vi "Finish.vi"   [LabVIEW 2018]
doc: "This VI is called just before exiting. It is expected to close I/O refnum, save collected data, etc."
uses:
  <vilib>/Rock Robotics/WPI/Utilities/WPI_GetSetVariantRefNum.vi
types:
  T1 = typedef "WPI_MotorControlDeviceRef.ctl" = cluster{"DeviceStatus":errorcluster, "Type":T2, "PWM":cluster{"PWM Channel":T3, "DeadBand":T4}, "CAN":cluster{"Device Number":u8, "SetOutput VI Ref":variant, "GetOutput VI Ref":variant, "Enable VI Ref":variant, "Disable VI Ref":variant, "Data":variant}, "Invert":bool, "DIO PWM":cluster{"PWM \"Enable\" Channel":T3, "DIOChannel":T5, "PWM Rate":dbl}}
  T2 = typedef "WPI_MotorControlType.ctl" = enum16{"PWM", "CAN", "DIO PWM"}
  T3 = typedef "FPGA_DIOPWMChannel.ctl" = enum8{"PWM 0", "PWM 1", "PWM 2", "PWM 3", "PWM 4", "PWM 5", "PWM 6", "PWM 7", "PWM 8", "PWM 9", "PWM MXP 0", "PWM MXP 1", "PWM MXP 2", "PWM MXP 3", "PWM MXP 4", "PWM MXP 5", "PWM MXP 6", "PWM MXP 7", "PWM MXP 8", "PWM MXP 9", "Invalid"}
  T4 = typedef "WPI_PWMDeadband.ctl" = cluster{"Name":string, "maxPositivePwm":i32, "minPositivePwm":i32, "centerPwm":i32, "maxNegativePwm":i32, "minNegativePwm":i32, "angularRange":u16}
  T5 = typedef "FPGA_DIOChannel.ctl" = enum8{"DIO 0", "DIO 1", "DIO 2", "DIO 3", "DIO 4", "DIO 5", "DIO 6", "DIO 7", "DIO 8", "DIO 9", "DIO MXP 0", "DIO MXP 1", "DIO MXP 2", "DIO MXP 3", "DIO MXP 4", "DIO MXP 5", "DIO MXP 6", "DIO MXP 7", "DIO MXP 8", "DIO MXP 9", "DIO MXP 10", "DIO MXP 11", "DIO MXP 12", "DIO MXP 13", "DIO MXP 14", "DIO MXP 15", "SPI Port CS1", "SPI Port CS2", "SPI Port CS3", "SPI Port MISO", "SPI Port MOSI", "Invalid"}
  T6 = typedef "WPI_SolenoidDevRef.ctl" = cluster{"DevStatus":errorcluster, "Pneumatics Control Module":u8, "Forward Solenoid Channel":T7, "Reverse Solenoid Channel":T7}
  T7 = typedef "WPI_SolenoidChannel.ctl" = enum8{"Solenoid 0", "Solenoid 1", "Solenoid 2", "Solenoid 3", "Solenoid 4", "Solenoid 5", "Solenoid 6", "Solenoid 7", "Invalid"}
  T8 = typedef "WPI_SwitchDevRef.ctl" = cluster{"DevStatus":errorcluster, "DIO Channel":T5, "CntIndex":T9, "Normally Closed":bool}
  T9 = typedef "FPGA_CounterCtrSystemIndex.ctl" = enum8{"Ctr 0", "Ctr 1", "Ctr 2", "Ctr 3", "Ctr 4", "Ctr 5", "Ctr 6", "Ctr 7", "Invalid"}
  T10 = typedef "WPI_JoystickDevRef.ctl" = cluster{"Device":T11}
  T11 = typedef "WPI_JoystickDeviceEnum.ctl" = enum16{"USB 0", "USB 1", "USB 2", "USB 3", "USB 4", "USB 5"}
  T12 = typedef "WPI_RobotDriveDevRef.ctl" = cluster{"DevStatus":errorcluster, "Motors[]":T1[], "Square Inputs":bool, "Max Output":dbl}
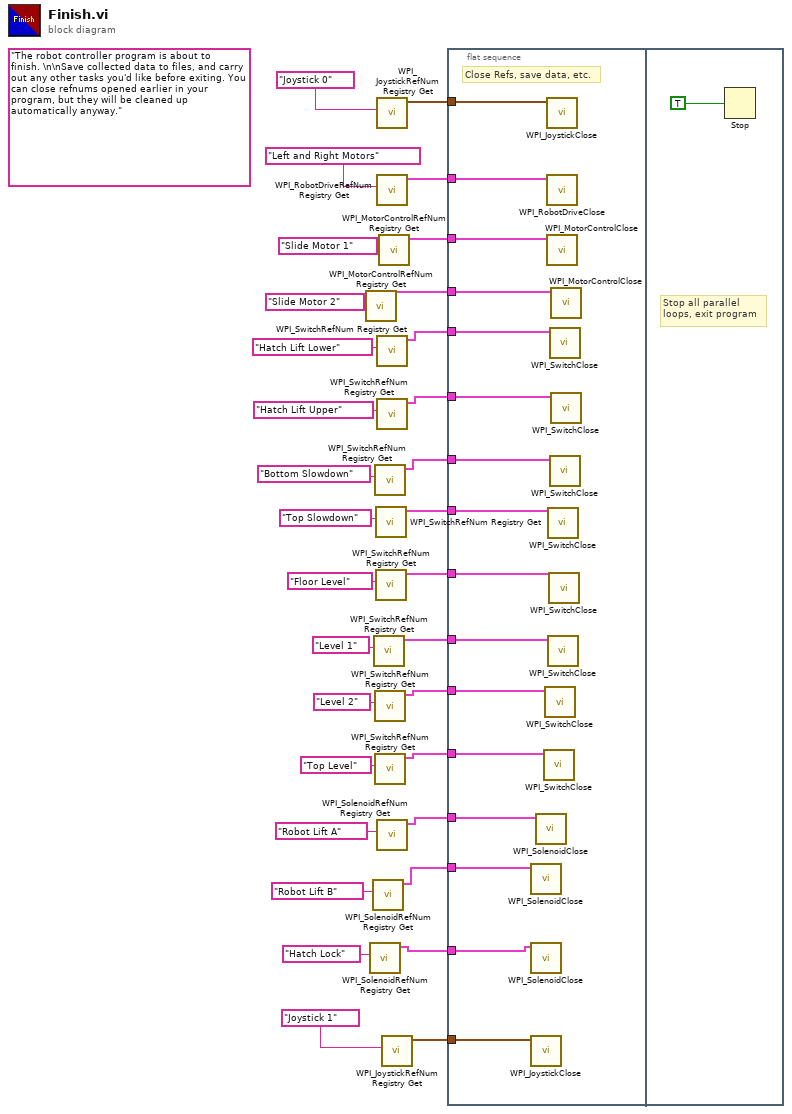
[diagram p0: block diagram]
diagram:
  (unwired) "The robot controller program is about to finish. \n\nSave collected data to files, and carry out any other tasks you'd like before exiting. You can close refnums opened earlier in your program, but they will be cleaned up automatically anyway."
  n1 = call <vilib>:"WPI_MotorControlRefNum Registry Get.vi"("refnum name"="Slide Motor 2") -> ("MotorControlDevRef"=w19:T1)  [unwired: 9 in, 1 out]
  n2 = call <vilib>:"WPI_SolenoidRefNum Registry Get.vi"("refnum name"="Hatch Lock") -> ("SolenoidDevRef"=w3:T6)  [unwired: 9 in, 1 out]
  n3 = call <vilib>:"WPI_SolenoidRefNum Registry Get.vi"("refnum name"="Robot Lift B") -> ("SolenoidDevRef"=w4:T6)  [unwired: 9 in, 1 out]
  n4 = call <vilib>:"WPI_SwitchRefNum Registry Get.vi"("refnum name"="Level 1") -> ("SwitchDevRef"=w24:T8)  [unwired: 9 in, 1 out]
  n5 = call <vilib>:"WPI_SwitchRefNum Registry Get.vi"("refnum name"="Bottom Slowdown") -> ("SwitchDevRef"=w11:T8)  [unwired: 9 in, 1 out]
  n6 = call <vilib>:"WPI_SwitchRefNum Registry Get.vi"("refnum name"="Level 2") -> ("SwitchDevRef"=w13:T8)  [unwired: 9 in, 1 out]
  n7 = call <vilib>:"WPI_SwitchRefNum Registry Get.vi"("refnum name"="Top Level") -> ("SwitchDevRef"=w12:T8)  [unwired: 9 in, 1 out]
  n8 = call <vilib>:"WPI_SwitchRefNum Registry Get.vi"("refnum name"="Top Slowdown") -> ("SwitchDevRef"=w28:T8)  [unwired: 9 in, 1 out]
  n9 = call <vilib>:"WPI_SwitchRefNum Registry Get.vi"("refnum name"="Floor Level") -> ("SwitchDevRef"=w25:T8)  [unwired: 9 in, 1 out]
  n10 = call <vilib>:"WPI_JoystickRefNum Registry Get.vi"("refnum name"="Joystick 0") -> ("JoystickDevRef"=w29:T10)  [unwired: 1 in, 9 out]
  n11 = call <vilib>:"WPI_RobotDriveRefNum Registry Get.vi"("refnum name"="Left and Right Motors") -> ("RobotDriveDevRef"=w30:T12)  [unwired: 1 in, 9 out]
  n12 = call <vilib>:"WPI_SwitchRefNum Registry Get.vi"("refnum name"="Hatch Lift Lower") -> ("SwitchDevRef"=w9:T8)  [unwired: 9 in, 1 out]
  n13 = call <vilib>:"WPI_SwitchRefNum Registry Get.vi"("refnum name"="Hatch Lift Upper") -> ("SwitchDevRef"=w10:T8)  [unwired: 9 in, 1 out]
  n14 = call <vilib>:"WPI_SolenoidRefNum Registry Get.vi"("refnum name"="Robot Lift A") -> ("SolenoidDevRef"=w5:T6)  [unwired: 9 in, 1 out]
  n15 = call <vilib>:"WPI_MotorControlRefNum Registry Get.vi"("refnum name"="Slide Motor 1") -> ("MotorControlDevRef"=w21:T1)  [unwired: 9 in, 1 out]
  n16 = call <vilib>:"WPI_JoystickRefNum Registry Get.vi"("refnum name"="Joystick 1") -> ("JoystickDevRef"=w1:T10)  [unwired: 1 in, 9 out]
  n17 = flat-sequence {
    tunnel: w30 -> [w48]
    tunnel: w29 -> [w47]
    tunnel: w28 -> [w46]
    tunnel: w25 -> [w45]
    tunnel: w24 -> [w44]
    tunnel: w21 -> [w43]
    tunnel: w19 -> [w42]
    tunnel: w13 -> [w41]
    tunnel: w12 -> [w40]
    tunnel: w11 -> [w39]
    tunnel: w10 -> [w38]
    tunnel: w9 -> [w37]
    tunnel: w5 -> [w36]
    tunnel: w4 -> [w35]
    tunnel: w3 -> [w34]
    tunnel: w1 -> [w33]
    frame #0 {
      # "Close Refs, save data, etc."
      n18 = call <vilib>:"WPI_SolenoidClose.vi"("SolenoidDevRef"=w35) -> ()  [unwired: 10 in, 1 out]
      n19 = call <vilib>:"WPI_SolenoidClose.vi"("SolenoidDevRef"=w34) -> ()  [unwired: 10 in, 1 out]
      n20 = call <vilib>:"WPI_JoystickClose.vi"("JoystickDevRef"=w33) -> ()  [unwired: 11 out]
      n21 = call <vilib>:"WPI_SolenoidClose.vi"("SolenoidDevRef"=w36) -> ()  [unwired: 10 in, 1 out]
      n22 = call <vilib>:"WPI_SwitchClose.vi"("SwitchDevRef"=w40) -> ()  [unwired: 10 in, 1 out]
      n23 = call <vilib>:"WPI_SwitchClose.vi"("SwitchDevRef"=w41) -> ()  [unwired: 10 in, 1 out]
      n24 = call <vilib>:"WPI_JoystickClose.vi"("JoystickDevRef"=w47) -> ()  [unwired: 11 out]
      n25 = call <vilib>:"WPI_RobotDriveClose.vi"("RobotDriveDevRef"=w48) -> ()  [unwired: 1 in, 10 out]
      n26 = call <vilib>:"WPI_MotorControlClose.vi"("MotorControlDevRef"=w43) -> ()  [unwired: 10 in, 1 out]
      n27 = call <vilib>:"WPI_SwitchClose.vi"("SwitchDevRef"=w46) -> ()  [unwired: 10 in, 1 out]
      n28 = call <vilib>:"WPI_SwitchClose.vi"("SwitchDevRef"=w44) -> ()  [unwired: 10 in, 1 out]
      n29 = call <vilib>:"WPI_SwitchClose.vi"("SwitchDevRef"=w45) -> ()  [unwired: 10 in, 1 out]
      n30 = call <vilib>:"WPI_SwitchClose.vi"("SwitchDevRef"=w37) -> ()  [unwired: 10 in, 1 out]
      n31 = call <vilib>:"WPI_SwitchClose.vi"("SwitchDevRef"=w39) -> ()  [unwired: 10 in, 1 out]
      n32 = call <vilib>:"WPI_MotorControlClose.vi"("MotorControlDevRef"=w42) -> ()  [unwired: 10 in, 1 out]
      n33 = call <vilib>:"WPI_SwitchClose.vi"("SwitchDevRef"=w38) -> ()  [unwired: 10 in, 1 out]
    }
    frame #1 {
      # "Stop all parallel\nloops, exit program"
      n34 = Stop(stop? (T)=TRUE ("Quit")) -> ()
    }
  }
